vi "Set Window Run-Time Position.vi"(8 "error in (no error)":errorcluster, 9 "Window Run-Time Position":T1=enum."Minimized", 10 "ProjectItem Refnum":refnum<vi>, 11 "NI_AB_API_EXE_Extensions in":refnum<class "NI_AB_API_EXE_Extensions.lvclass">) -> (0 "error out":errorcluster, 3 "NI_AB_API_EXE_Extensions out":refnum<class "NI_AB_API_EXE_Extensions.lvclass">)   [LabVIEW 2021, in "NI_AB_API_EXE_Extensions.lvclass"]
uses:
  NI_AB_API_EXE_Extensions.lvclass
  NI_AB_API_EXE_Extensions.lvclass/NI_AB_API_EXE_Extensions.ctl
  <vilib>/AppBuilder/AB_API/Build/NI_AB_API_Build.lvclass
  <vilib>/AppBuilder/AB_Classes/EXE/AB_EXE.lvclass
  <vilib>/AppBuilder/AB_Classes/Build/AB_Build.lvclass
  <vilib>/AppBuilder/AB_Classes/Source/AB_Source.lvclass
  <vilib>/AppBuilder/AB_Source_Property_Type.ctl
  <vilib>/AppBuilder/AB_Source_Properties.ctl
  <vilib>/ErrorRing/Error Ring.xnode
  <vilib>/Utility/error.llb/Error Cluster From Error Code.vi
  C:/Program Files/National Instruments/LabVIEW 2021/vi.lib/AppBuilder/AB_API/EXE/NI_AB_API_EXE.lvclass
  C:/Program Files/National Instruments/LabVIEW 2021/vi.lib/AppBuilder/AB_API/Application/NI_AB_API_Application.lvclass
  C:/Program Files/National Instruments/LabVIEW 2021/vi.lib/AppBuilder/AB_API/Targetfile/NI_AB_API_Targetfile.lvclass
  C:/Program Files/National Instruments/LabVIEW 2021/vi.lib/AppBuilder/AB_API/Build/NI_AB_API_Build.lvclass
  C:/Program Files/National Instruments/LabVIEW 2021/vi.lib/AppBuilder/AB_Classes/Application/AB_Application.lvclass
  C:/Program Files/National Instruments/LabVIEW 2021/vi.lib/AppBuilder/AB_Classes/TargetFile/AB_Targetfile.lvclass
  C:/Program Files/National Instruments/LabVIEW 2021/vi.lib/AppBuilder/AB_Classes/Build/AB_Build.lvclass
  C:/Program Files/National Instruments/LabVIEW 2021/vi.lib/AppBuilder/AB_Classes/EXE/AB_EXE.lvclass
  <vilib>/AppBuilder/AB_Source_Property_WindowRunTimePosition.ctl
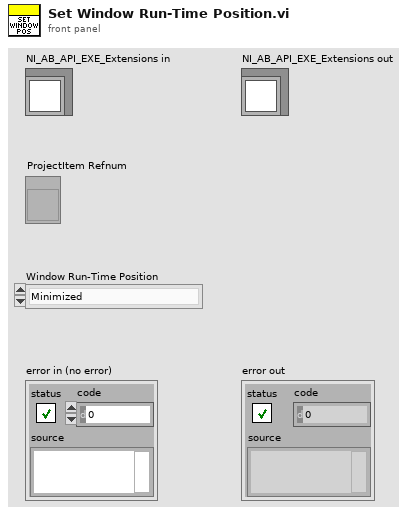
[diagram p1: front panel]
types:
  T1 = typedef "AB_Source_Property_WindowRunTimePosition.ctl" = enum16{"Unchanged", "Centered", "Maximized", "Minimized"}
  T2 = typedef "AB_Source_Properties.ctl" = cluster{"sourcePropertyType":T3, "value":variant}
  T3 = typedef "AB_Source_Property_Type.ctl" = enum16{"Remove block diagram", "Remove front panel", "Password", "Window has title bar", "Show menu bar", "Show vertical scroll bar", "Show horizontal scroll bar", "Show toolbar", "Show Abort button", "Show fp when called", "Window behavior", "Allow user to close window", "Window run-time position", "Run when opened", "Allow debugging", "Auto error handling", "Generate guard code", "Use stack variables", "Expression folding", "Integer only", "Inline subVI"}
  T4 = typedef "AB_Source.ctl" = cluster{"path":path, "itemID":string, "parentIndex":i32, "sourceInclusion":T5, "destinationIndex":i32, "properties":T2[], "newName":string, "lvfile":bool, "valid":bool, "eng_inBuild":bool, "eng_isNonVILink":bool, "Amalgamation":bool, "Amalgamation Piece":bool, "eng_delimitedName":string, "preventRename":bool}
  T5 = typedef "AB_Source_Inclusion.ctl" = enum16{"IncludeIfReferenced", "Include", "Exclude", "TopLevel"}
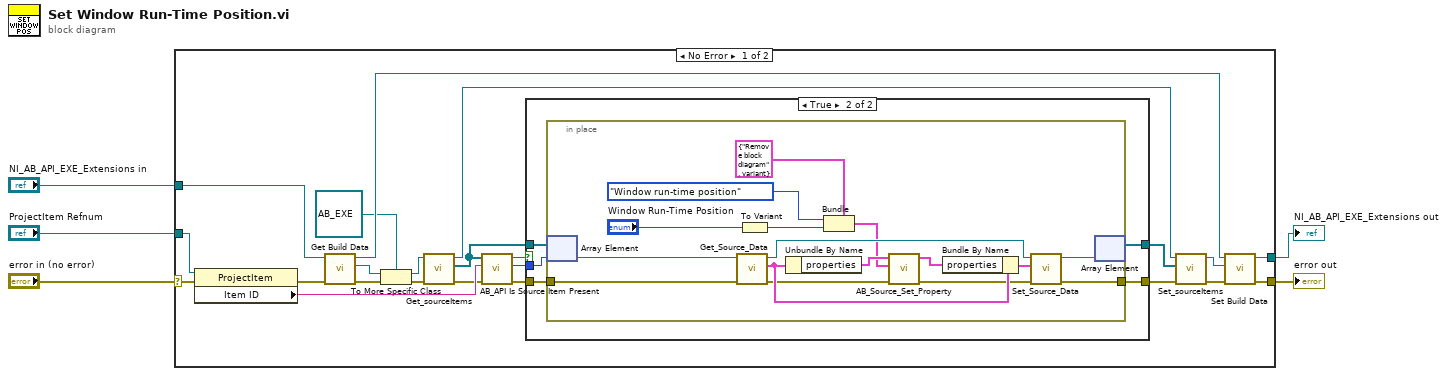
[diagram p0: block diagram]
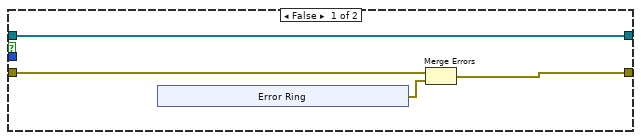
[diagram p2: hidden frame]
diagram:
  n1 = case shown="No Error" "error in (no error)" {
    selector: "error in (no error)" -> [w7 w60]
    tunnel: [w23 w60] -> w4
    tunnel: [w24 w59] -> w2
    tunnel: "NI_AB_API_EXE_Extensions in" -> [w25 w59]
    tunnel: "ProjectItem Refnum" -> [w8 _]
    frame No Error {
      n2 = property class="ProjectItem"(reference=w8, error in=w7) -> (error out=w6:errorcluster, "Item ID"=w16:string)  [unwired: 1 out]
      n3 = call <vilib>:"Get Build Data.vi"("error in (no error)"=w6, "NI_AB_API_Build in"=w25) -> ("error out"=w26:errorcluster, "AB_Build.lvclass"=w27:refnum<class "AB_Build.lvclass">, "NI_AB_API_Build in"=w28:refnum<class "NI_AB_API_EXE_Extensions.lvclass">)  [unwired: 7 in]
      n4 = To More Specific Class(target class=refnum<class "AB_EXE.lvclass"> refnum ("AB_EXE.lvclass"), reference=w27, error in=w26) -> (specific class reference=w20:refnum<class "AB_EXE.lvclass">, error out=w21:errorcluster)
      n5 = call <vilib>:"Get_sourceItems.vi"("error in (no error)"=w21, "Class in"=w20) -> ("error out"=w15:errorcluster, "sourceItems"=w11:refnum<class "AB_Source.lvclass">[], "Class out"=w17:refnum<class "AB_EXE.lvclass">)  [unwired: 7 out]
      n6 = call <vilib>:"AB_API Is Source Item Present.vi"("error in"=w15, "item ID"=w16, "source items"=w11) -> ("error out"=w12:errorcluster, "index"=w13:i32, "source item present?"=w14:bool)  [unwired: 3 in, 3 out]
      n7 = case shown="True" w14 {
        tunnel: w13 -> [_ w41]
        tunnel: w12 -> [w31 w40]
        tunnel: w11 -> [w32 w42]
        tunnel: [w30 w39] -> w9
        tunnel: [w32 w38] -> w10
        frame False {
          n8 = xnode "Error Ring"() -> ("error out"=w29:errorcluster)
          n9 = Merge Errors(w31, w29) -> (w30:errorcluster)
        }
        frame True {
          n10 = in-place {
            in-place-border: w40 -> [w56]
            in-place-border: [w50] -> w39
            n11 = in-place-array #1(w42, w41) -> (w58:refnum<class "AB_Source.lvclass">)
            n12 = call <vilib>:"Get_Source_Data.vi"("error in (no error)"=w56, "Class in"=w58) -> ("error out"=w49:errorcluster, "data"=w55:T4, "Class out"=w57:refnum<class "AB_Source.lvclass">)  [unwired: 7 in]
            n13 = To Variant(anything="Window Run-Time Position") -> (Variant=w45:variant)
            n14 = Unbundle By Name(w55) -> ("properties"=w54:T2[])
            n15 = Bundle(cluster=T2 {"sourcePropertyType"=enum."Remove block diagram", "value"=variant} ("sourceProperties"), "sourcePropertyType"=AB_Source_Property_Type."Window run-time position", "value"=w45) -> (w44:T2)
            n16 = call <vilib>:"AB_Source_Set_Property.vi"("error in (no error)"=w49, "sourceProperty"=w44, "sourceProperties in"=w54) -> ("error out"=w48:errorcluster, "sourceProperties out"=w53:T2[])  [unwired: 6 in, 1 out]
            n17 = Bundle By Name(cluster=w55, "properties"=w53) -> (w52:T4)
            n18 = call <vilib>:"Set_Source_Data.vi"("error in (no error)"=w48, "data"=w52, "Class in"=w57) -> ("error out"=w50:errorcluster, "Class out"=w51:refnum<class "AB_Source.lvclass">)  [unwired: 7 in]
            n19 = in-place-array #1(w51) -> (w38:refnum<class "AB_Source.lvclass">[])  [unwired: 1 out]
          }
        }
      }
      n20 = call <vilib>:"Set_sourceItems.vi"("error in (no error)"=w9, "sourceItems"=w10, "Class in"=w17) -> ("error out"=w19:errorcluster, "Class out"=w18:refnum<class "AB_EXE.lvclass">)  [unwired: 7 out]
      n21 = call <vilib>:"Set Build Data.vi"("error in (no error)"=w19, "AB_Build.lvclass"=w18, "NI_AB_API_Build in"=w28) -> ("error out"=w23:errorcluster, "NI_AB_API_Build in"=w24:refnum<class "NI_AB_API_EXE_Extensions.lvclass">)  [unwired: 7 in]
    }
    frame Error {
    }
  }
  "error out" <- w4
  "NI_AB_API_EXE_Extensions out" <- w2
